vi "S1500_S7Com_RESP(SubVI).vi"(9 "PDU_In":T5 format="X%02x", 10 "Seq# In":u16, 11 "Transport Size In":T1 items=["BIT"=1, "BYTE"=2, "CHAR"=3, "WORD"=4, "INT"=5, "DWORD"=6, "DINT"=7, "REAL"=8]) -> (1 "Output_Data":T4, 2 "Error":bool)   [LabVIEW 2018]
doc: "Decodes the S7 Protocol Response."
uses:
  S1500_test_S7Com_HexByteArray.ctl
  S1500_S7Com_HexByte.ctl
  S1500_S7Com_Data_Array.ctl
  S1500_S7Com_Function.ctl
  S1500_S7Com_Transport_Size.ctl
panel:
  out "Return Code not 0Xff":bool
  out "Error not 0X00":bool
  out "Data Length 4":u16 format="X%02x"
  out "S7_Function":T2=4 items=["Read"=4, "Write"=5]
  out "Return Code":u8 format="%02x"
  out "Item Count":u8 format="%02x"
  out "Error Code":u16 format="%02x"
  out "Data Length":u16 format="%02x"
  out "Param Length":T3 format="%02x"
  out "Seq# Mismatch":bool
  out "Not Response":bool
  out "Not S7 Comm":bool
  out "Seq# Out":u16
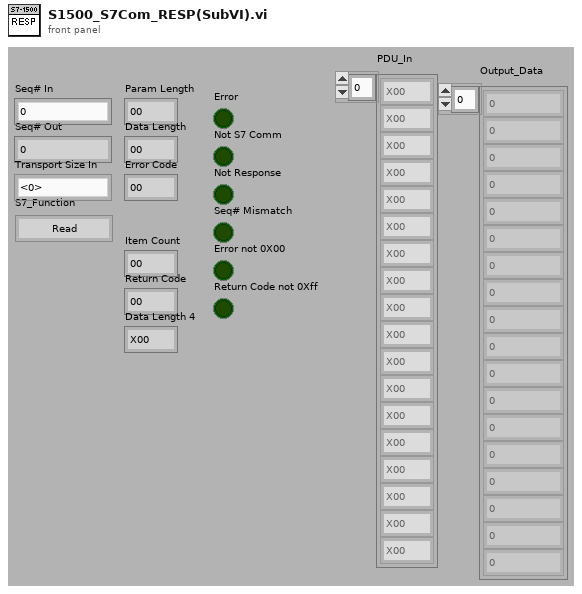
[diagram p1: front panel]
types:
  T1 = typedef "S1500_S7Com_Transport_Size.ctl" = u8
  T2 = typedef "S1500_S7Com_Function.ctl" = u8
  T3 = typedef "S1500_S7Com_HexByte.ctl" = u8
  T4 = typedef "S1500_S7Com_Data_Array.ctl" = i32[]
  T5 = typedef "S1500_test_S7Com_HexByteArray.ctl" = T3[]
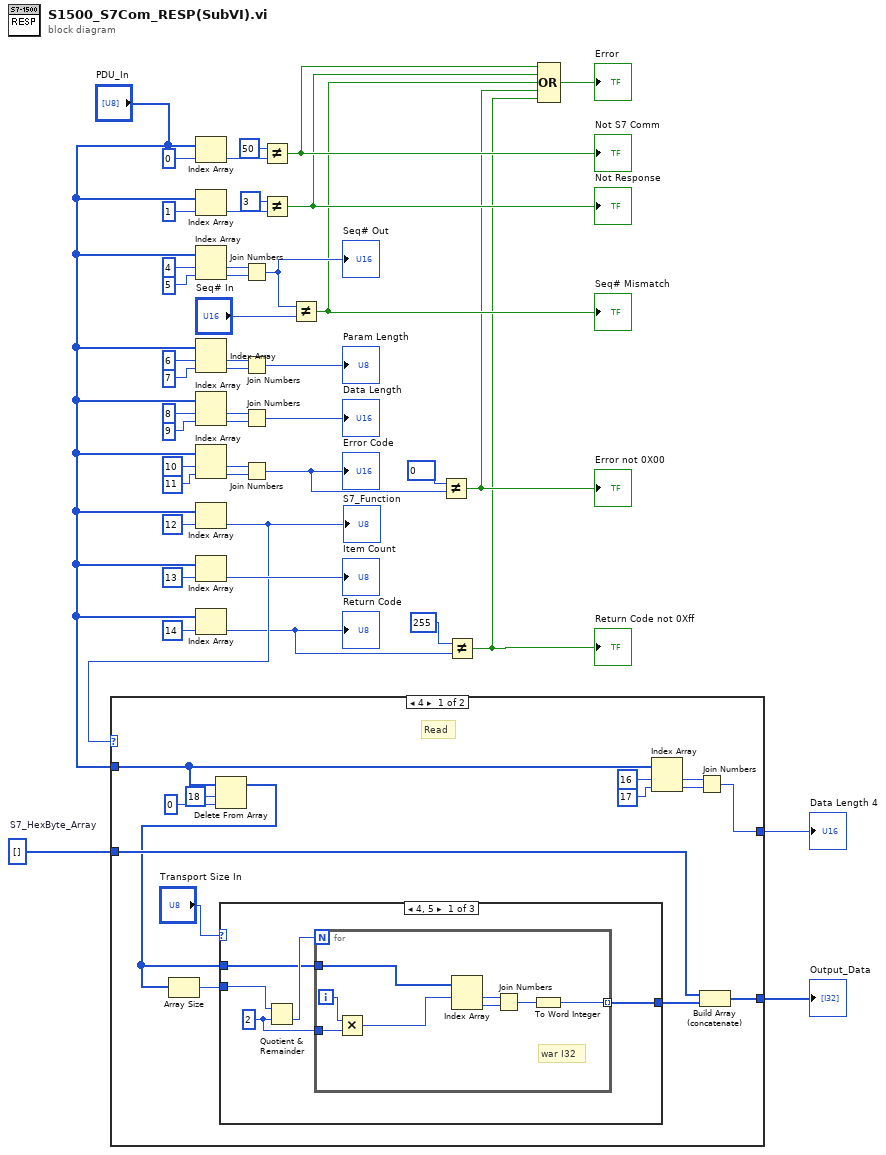
[diagram p0: block diagram]
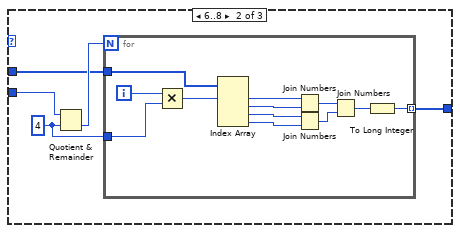
[diagram p2: hidden frame]
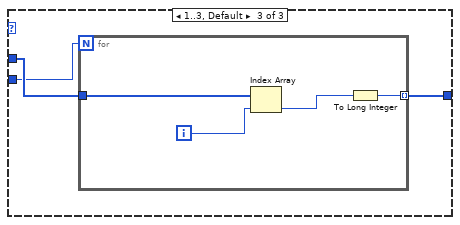
[diagram p3: hidden frame]
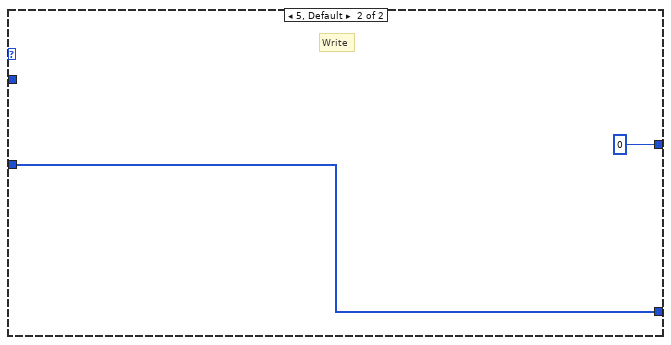
[diagram p4: hidden frame]
diagram:
  w6 = T5 []  # S7_HexByte_Array
  n1 = Index Array(array="PDU_In", index=0) -> (element=w43:T3)
  n2 = Index Array(array="PDU_In", index=1) -> (element=w39:T3)
  n3 = Index Array(array="PDU_In", index #1=4, index #2=5) -> (element #1=w36:T3, element #2=w37:T3)
  n4 = Index Array(array="PDU_In", index #1=6, index #2=7) -> (element #1=w30:T3, element #2=w31:T3)
  n5 = Index Array(array="PDU_In", index #1=8, index #2=9) -> (element #1=w25:T3, element #2=w26:T3)
  n6 = Index Array(array="PDU_In", index #1=10, index #2=11) -> (element #1=w21:T3, element #2=w22:T3)
  n7 = Index Array(array="PDU_In", index=12) -> (element=w12:T3)
  "S7_Function" <- w12
  n8 = case shown="4" w12 {
    tunnel: "PDU_In" -> [w49 _]
    tunnel: [w51 w97] -> w10
    tunnel: [w55 u16 0] -> w3
    tunnel: w6 -> [w52 w97]
    frame 4 {
      # "Read"
      n9 = Delete From Array(array=w49, length=18 ("index"), index=0) -> (array with subset deleted=w46:T5)  [unwired: 1 out]
      n10 = Array Size(array=w46) -> (size(s)=w53:i32)
      n11 = case shown="4, 5" "Transport Size In" {
        tunnel: [w61 w74 w92] -> w50
        tunnel: w53 -> [w63 w76 w90]
        tunnel: w46 -> [w62 w75 w91]
        frame 4, 5 {
          w60 = 2
          n12 = Quotient & Remainder(x=w63, y=w60) -> (floor(x/y)=w64:i32)  [unwired: 1 out]
          n13 = for {
            N: w64 -> [_]
            tunnel: w62 -> [w72]
            tunnel: [w68] -> w61 mode=indexing
            tunnel: w60 -> [w67]
            i -> [w66]
            # "war I32"
            n14 = Multiply(x=w66, y=w67) -> (x*y=w65:i32)
            n15 = Index Array(array=w72, index #1=w65) -> (element #1=w70:T3, element #2=w71:T3)  [unwired: 1 in]
            n16 = Join Numbers(hi=w70, lo=w71) -> ((hi.lo)=w69:u16)
            n17 = To Word Integer(number=w69) -> (16bit integer=w68:i16)
          }
        }
        frame 6..8 {
          w73 = 4
          n18 = Quotient & Remainder(x=w76, y=w73) -> (floor(x/y)=w77:i32)  [unwired: 1 out]
          n19 = for {
            N: w77 -> [_]
            tunnel: w75 -> [w89]
            tunnel: [w86] -> w74 mode=indexing
            tunnel: w73 -> [w85]
            i -> [w84]
            n20 = Multiply(x=w84, y=w85) -> (x*y=w78:i32)
            n21 = Index Array(array=w89, index #1=w78) -> (element #1=w87:T3, element #2=w88:T3, element #3=w83:T3, element #4=w82:T3)  [unwired: 3 in]
            n22 = Join Numbers(hi=w87, lo=w88) -> ((hi.lo)=w81:u16)
            n23 = Join Numbers(hi=w83, lo=w82) -> ((hi.lo)=w80:u16)
            n24 = Join Numbers(hi=w81, lo=w80) -> ((hi.lo)=w79:u32)
            n25 = To Long Integer(number=w79) -> (32bit integer=w86:i32)
          }
        }
        frame 1..3, Default {
          n26 = for {
            N: w90 -> [_]
            tunnel: [w96] -> w92 mode=indexing
            tunnel: w91 -> [w95]
            i -> [w93]
            n27 = Index Array(array=w95, index=w93) -> (element=w94:T3)
            n28 = To Long Integer(number=w94) -> (32bit integer=w96:i32)
          }
        }
      }
      n29 = Index Array(array=w49, index #1=16, index #2=17) -> (element #1=w59:T3, element #2=w58:T3)
      n30 = Join Numbers(hi=w59, lo=w58) -> ((hi.lo)=w55:u16)
      n31 = Build Array (concatenate)(w52, w50) -> (w51:i32[])
    }
    frame 5, Default {
      # "Write"
    }
  }
  "Output_Data" <- w10
  "Data Length 4" <- w3
  n32 = Index Array(array="PDU_In", index=13) -> (element=→"Item Count":T3)
  n33 = Index Array(array="PDU_In", index=14) -> (element=w5:T3)
  "Return Code" <- w5
  n34 = Join Numbers(hi=w36, lo=w37) -> ((hi.lo)=w35:u16)
  "Seq# Out" <- w35
  n35 = Join Numbers(hi=w30, lo=w31) -> ((hi.lo)=→"Param Length":u16)
  n36 = Join Numbers(hi=w25, lo=w26) -> ((hi.lo)=→"Data Length":u16)
  n37 = Join Numbers(hi=w21, lo=w22) -> ((hi.lo)=w8:u16)
  "Error Code" <- w8
  n38 = Not Equal?(x=u8 50, y=w43) -> (x != y?=w15:bool)
  "Not S7 Comm" <- w15
  n39 = Not Equal?(x=u8 3, y=w39) -> (x != y?=w14:bool)
  "Not Response" <- w14
  n40 = Not Equal?(x=w35, y="Seq# In") -> (x != y?=w13:bool)
  "Seq# Mismatch" <- w13
  n41 = Not Equal?(x=u16 0, y=w8) -> (x != y?=w7:bool)
  "Error not 0X00" <- w7
  n42 = Not Equal?(x=u8 255, y=w5) -> (x != y?=w1:bool)
  "Return Code not 0Xff" <- w1
  n43 = Compound Arithmetic op=OR(w15, w14, w13, w7, w1) -> (→"Error":bool)
